vi "read parameters limits.vi"(8 "error in (no error)":errorcluster, 11 "Simulated_CCD_Camera in":refnum<class "Simulated Camera.lvclass">) -> (0 "error out":errorcluster, 2 "limit values spreadsheet":string[][](array[string]), 3 "Simulated_CCD_Camera out":refnum<class "Simulated Camera.lvclass">)   [LabVIEW 2018, in "Simulated Camera.lvclass"]
uses:
  Simulated Camera.lvclass
  Simulated Camera.lvclass/Simulated Camera.ctl
  <vilib>/Utility/file.llb/Read Delimited Spreadsheet (string).vi
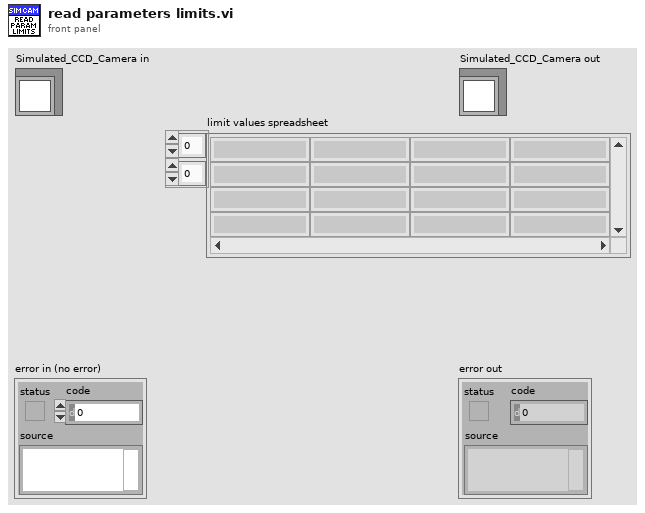
[diagram p1: front panel]
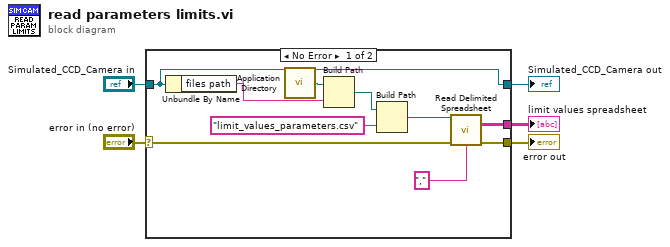
[diagram p0: block diagram]
diagram:
  n1 = case shown="No Error" "error in (no error)" {
    selector: "error in (no error)" -> [w14 w17]
    tunnel: [w13 w17] -> w4
    tunnel: [w11 w16] -> w2
    tunnel: "Simulated_CCD_Camera in" -> [w11 w16]
    tunnel: [w12 _] -> w1
    frame No Error {
      n2 = Unbundle By Name(w11) -> ("files path"=w10:string)
      n3 = call <vilib>:"Application Directory.vi"() -> ("Application Directory"=w9:path)
      n4 = Build Path(base path=w9, name or relative path=w10) -> (appended path=w8:path)
      n5 = Build Path(base path=w8, name or relative path="limit_values_parameters.csv") -> (appended path=w6:path)
      n6 = call-poly <vilib>:"Read Delimited Spreadsheet.vi"("file path (dialog if empty)"=w6, "error in (no error)"=w14, "delimiter (\\t)"="," ("delimiter (\\t)")) -> ("all rows"=w12:string[][], "error out"=w13:errorcluster)  [unwired: 7 in, 4 out]
    }
    frame Error {
    }
  }
  "error out" <- w4
  "Simulated_CCD_Camera out" <- w2
  "limit values spreadsheet" <- w1
